vi "DIst to Ticks.vi"(11 "x":dbl) -> (3 "Numeric":dbl)   [LabVIEW 2016]
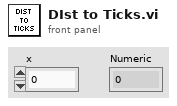
[diagram p1: front panel]
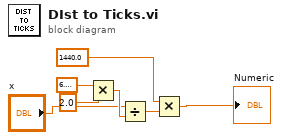
[diagram p0: block diagram]
diagram:
  n1 = Multiply(x=6.283185307179586, y=2.0) -> (x*y=w4:dbl)
  n2 = Divide(x="x", y=w4) -> (x/y=w5:dbl)
  n3 = Multiply(x=1440.0, y=w5) -> (x*y=→"Numeric":dbl)
